vi "Test_ConstructTransport_InvalidRefnum_Error.vi"(8 "error in (no error)":errorcluster, 11 "TestCase in":refnum<class "TestMCListboxItemNamesBinding.lvclass">) -> (0 "error out":errorcluster, 3 "TestCase out":refnum<class "TestMCListboxItemNamesBinding.lvclass">)   [LabVIEW 2017, in "TestMCListboxItemNamesBinding.lvclass"]
uses:
  TestMCListboxItemNamesBinding.lvclass
  Source/Concrete/MCListboxItemNamesBinding/MCListboxItemNamesBinding.lvclass/MCListboxItemNamesBinding.ctl
  <vilib>/Utility/error.llb/Error Cluster From Error Code.vi
  Source/Concrete/MCListboxItemNamesBinding/MCListboxItemNamesBinding.lvclass
panel:
  out "Return Error":errorcluster
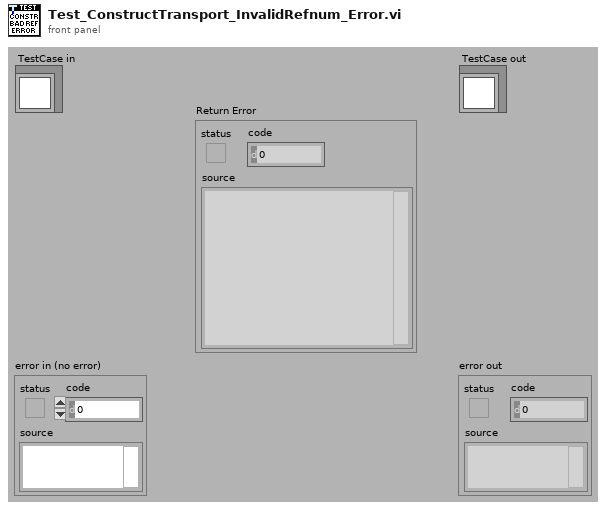
[diagram p1: front panel]
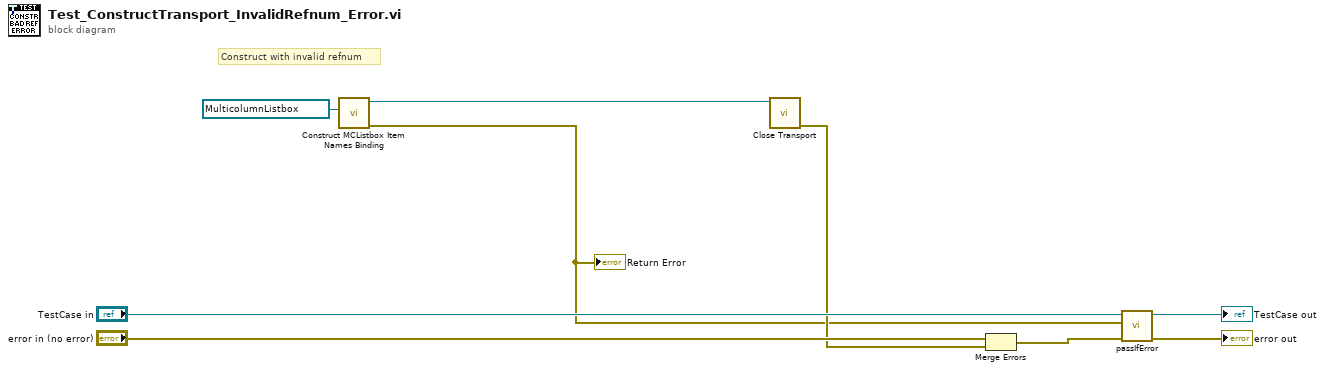
[diagram p0: block diagram]
diagram:
  # "Construct with invalid refnum"
  n1 = call "Construct MCListbox Item Names Binding.vi"("MCListbox Refnum"=refnum<vi> refnum) -> ("error out"=w1:errorcluster, "MCListboxItemNamesBinding"=w2:refnum<class "MCListboxItemNamesBinding.lvclass">)  [unwired: 9 in]
  "Return Error" <- w1
  n2 = call-dynamic "Close Transport.vi"("ITransport in"=w2) -> ("error out"=w4:errorcluster)  [unwired: 10 in]
  n3 = Merge Errors("error in (no error)", w4) -> (w5:errorcluster)
  n4 = call-dynamic "passIfError.vi"("error in (no error)"=w5, "error"=w1, "TestCase in"="TestCase in") -> ("error out"=→"error out":errorcluster, "TestCase out"=→"TestCase out":refnum<class "TestMCListboxItemNamesBinding.lvclass">)  [unwired: 7 in]
